vi "xiC - Tree_MenuActivation.vi"(6 "Menu Refnum":refnum<k9>, 8 "error in (no error)":errorcluster, 11 "Attributes In":T1) -> (0 "error out":errorcluster, 3 "Attributes Out":T1)   [LabVIEW 2015]
uses:
  xiC - Attributes.ctl
  C:/GIT/Cameras3.x/Integrations/Labview/xiLib/xiLIB_32bit/xiLIB/xiCamLib/API/x86/xiApi.NET.dll
  xiLIB_32bit/xiLIB/xiCamLib/API/x86/xiApi.NET.dll
  xiC - TreeDisplayType.ctl
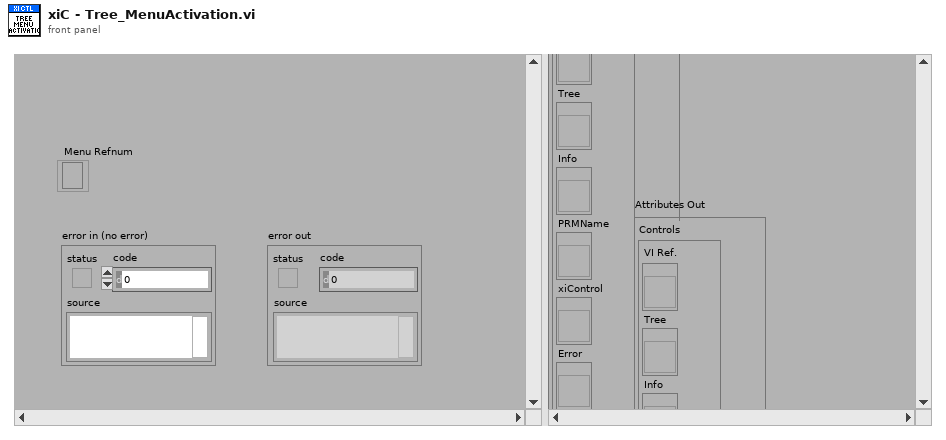
[diagram p1: front panel]
types:
  T1 = typedef "xiC - Attributes.ctl" = cluster{"Controls":cluster{"VI Ref.":refnum<vi>, "Tree":refnum<vi>, "Info":refnum<vi>, "PRMName":refnum<vi>, "xiControl":refnum<vi>, "Error":refnum<vi>, "SW_TRG":refnum<vi>, "ImageDisplay":refnum<vi>}, "Variables":cluster{"ProcessQ.":refnum<queue>, "Data":bool, "xiCam":refnum<k24>, "Tree_Display_Type":T2}}
  T2 = typedef "xiC - TreeDisplayType.ctl" = enum16{"DEFAULT", "HIDE_MAX_MIN"}
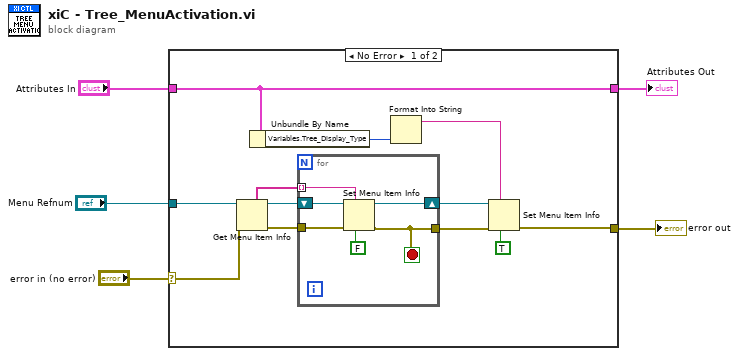
[diagram p0: block diagram]
diagram:
  n1 = case shown="No Error" "error in (no error)" {
    selector: "error in (no error)" -> [w15 w25]
    tunnel: [w6 w25] -> w4
    tunnel: "Attributes In" -> [w17 w24]
    tunnel: [w17 w24] -> w2
    tunnel: "Menu Refnum" -> [w16 _]
    frame No Error {
      n2 = Get Menu Item Info(8:w15, 11:w16) -> (0:w12:errorcluster, 3:w14:refnum<k9>, 5:w13:string[])  [unwired: 1 in, 4 out]
      n3 = Unbundle By Name(w17) -> ("Variables.Tree_Display_Type"=w9:T2)
      n4 = for {
        tunnel: [w18] -> w11
        shift-right: [w22] -> w10
        shift-left: w14 -> [w23]
        tunnel: w13 -> [w21] mode=indexing
        tunnel: w12 -> [w19]
        stop <- w18 stop-if-true
        n5 = Set Menu Item Info(6:FALSE ("checked"), 7:w21, 8:w19, 11:w23) -> (0:w18:errorcluster, 3:w22:refnum<k9>)  [unwired: 3 in]
      }
      n6 = Format Into String(w9) -> (resulting string=w8:string)  [unwired: 3 in, 1 out]
      n7 = Set Menu Item Info(6:TRUE ("checked"), 7:w8, 8:w11, 11:w10) -> (0:w6:errorcluster)  [unwired: 3 in, 1 out]
    }
    frame Error {
    }
  }
  "error out" <- w4
  "Attributes Out" <- w2
